vi "Begin.vi"(11 "Image Size":T1=enum."160x120") -> (0 "error out":errorcluster)   [LabVIEW 2012]
doc: "Called before other user functions, this VI is expected to open initial I/O refnums, load in file data, and do all program initialization. Notice that the <B>error out</B> terminal is simply used for data flow. Wiring it to other structures or subVIs ensures that this VI runs first."
uses:
  <vilib>/Rock Robotics/WPI/Camera/WPI_CameraImageSize.ctl
  <vilib>/Rock Robotics/SystemInterfaces/DIO/FPGA_DIOPWMChannel.ctl
  <vilib>/Rock Robotics/WPI/Camera/WPI_CameraWhite Balance Values.ctl
  <vilib>/Rock Robotics/WPI/Camera/WPI_CameraExposure Values.ctl
  <vilib>/Rock Robotics/WPI/Camera/WPI_CameraFrameRate.ctl
  <vilib>/Rock Robotics/WPI/SafetyOutput/WPI_SafetyOutputConfigMenu.ctl
  <vilib>/Rock Robotics/WPI/DriverStation/WPI_DriverStationRobotMode2.ctl
  <vilib>/Rock Robotics/WPI/Joystick/WPI_JoystickDeviceEnum.ctl
  <vilib>/Rock Robotics/SystemInterfaces/DIO/FPGA_DIORelayChannel.ctl
  <vilib>/Rock Robotics/SystemInterfaces/DIO/FPGA_DIOChannel.ctl
  <vilib>/Rock Robotics/WPI/Encoder/WPI_EncoderType.ctl
  <vilib>/Rock Robotics/SystemInterfaces/Typedef/FPGA_TypedefDigitalModule.ctl
  Program Files (x86)/National Instruments/LabVIEW 2012/examples/FRC/I2C/ADXL345 I2C/Driver/ADXL345 I2C Range.ctl
  <vilib>/Rock Robotics/WPI/RobotDrive/WPI_RobotDriveOpen2MotorWithJaguar.vi
  Robot Global Data.vi
  <vilib>/Rock Robotics/WPI/MotorControl/WPI_MotorControlOpen Jaguar.vi
  <vilib>/Rock Robotics/WPI/Counter/WPI_CounterDigitalInputToDigitalSource.vi
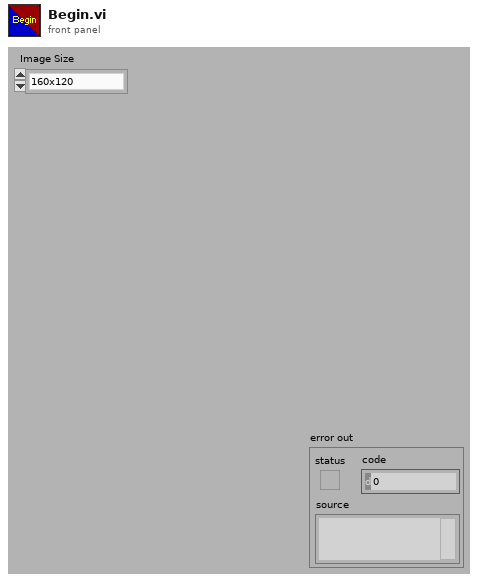
[diagram p1: front panel]
types:
  T1 = typedef "WPI_CameraImageSize.ctl" = enum16{"640x480", "320x240", "160x120"}
  T2 = typedef "FPGA_DIOPWMChannel.ctl" = enum8{"PWM 1", "PWM 2", "PWM 3", "PWM 4", "PWM 5", "PWM 6", "PWM 7", "PWM 8", "PWM 9", "PWM 10", "Invalid"}
  T3 = typedef "ADXL345 I2C Range.ctl" = u8
  T4 = typedef "FPGA_TypedefDigitalModule.ctl" = enum16{"Digital Module 1", "Digital Module 2"}
  T5 = typedef "WPI_EncoderType.ctl" = enum16{"1x", "2x", "4x"}
  T6 = typedef "FPGA_DIOChannel.ctl" = enum8{"DIO 1", "DIO 2", "DIO 3", "DIO 4", "DIO 5", "DIO 6", "DIO 7", "DIO 8", "DIO 9", "DIO 10", "DIO 11", "DIO 12", "DIO 13", "DIO 14", "Invalid"}
  T7 = typedef "FPGA_DIORelayChannel.ctl" = enum8{"Relay 1", "Relay 2", "Relay 3", "Relay 4", "Relay 5", "Relay 6", "Relay 7", "Relay 8", "Invalid"}
  T8 = typedef "WPI_JoystickDeviceEnum.ctl" = enum16{"USB 1", "USB 2", "USB 3", "USB 4", "Kinect 1", "Kinect 2"}
  T9 = typedef "WPI_DriverStationRobotMode2.ctl" = enum16{"Autonomous Disabled", "Autonomous Enabled", "Teleop Disabled", "Teleop Enabled", "Timeout", "Finish", "Test Disabled", "Test Enabled"}
  T10 = typedef "WPI_SafetyOutputConfigMenu.ctl" = enum16{"Enable", "Disable"}
  T11 = typedef "WPI_CameraFrameRate.ctl" = u32
  T12 = typedef "WPI_CameraExposure Values.ctl" = enum16{"Auto", "Flicker-free 50 Hz", "Flicker-free 60 Hz", "Hold current"}
  T13 = typedef "WPI_CameraWhite Balance Values.ctl" = enum16{"Auto", "Fixed indoor", "Fixed outdoor 1", "Fixed outdoor 2", "Fixed fluorescent 1", "Fixed fluorescent 2", "Hold current"}
  T14 = typedef "WPI_DigitalInputDevRef.ctl" = cluster{"DevStatus":errorcluster, "DIO Channel":T6, "Digital Module":T4}
  T15 = typedef "WPI_RelayDevRef.ctl" = cluster{"DevStatus":errorcluster, "Relay Channel":T7, "Digital Module":T4, "Relay Direction":T16}
  T16 = typedef "WPI_RelayDirection.ctl" = enum16{"Both directions", "Forward only", "Reverse only"}
  T17 = typedef "WPI_CameraDevRef.ctl" = cluster{"Camera Address":string, "CameraStatus":errorcluster, "Acquire Image Notifier":refnum<notifier>}
  T18 = typedef "WPI_JoystickDevRef.ctl" = cluster{"Device":T8}
  T19 = typedef "WPI_RobotDriveDevRef.ctl" = cluster{"DevStatus":errorcluster, "Motors[]":T20[], "Square Inputs":bool, "Max Output":dbl, "Isochronous":bool}
  T20 = typedef "WPI_MotorControlDeviceRef.ctl" = cluster{"DeviceStatus":errorcluster, "Type":enum16{"PWM", "CAN"}, "PWM":cluster{"Digital Module":T4, "PWM Channel":T2, "DeadBand":T21}, "CAN":cluster{"Device Number":u8, "Control Mode":T22, "Semaphore":T23, "Max Vout":dbl}, "Invert":bool, "TransformRef":T24, "InvTransformRef":T24}
  T21 = typedef "WPI_PWMDeadband.ctl" = cluster{"Name":string, "maxPositivePwm":i32, "minPositivePwm":i32, "centerPwm":i32, "maxNegativePwm":i32, "minNegativePwm":i32, "angularRange":u16}
  T22 = typedef "WPI_CANJaguar_ControlMode.ctl" = enum8{"Percent VBus", "Current", "Speed", "Position", "Voltage"}
  T23 = typedef "Semaphore RefNum" = refnum<k1>
  T24 = typedef "WPI_PWMTransform_ConPane.ctl" = refnum<vi>
  T25 = typedef "FPGA_CounterEncoderSourceConvertionLVSourceType.ctl" = cluster{"DevStatus":errorcluster, "AnalogTriggerMode?":bool, "DigitalMode":cluster{"Digital Module":T4, "DIO Channel":T26}, "AnalogTriggerMode":cluster{"AnalogTriggerIndex":T27, "OutputType":T28}}
  T26 = typedef "FPGA_DIODigitalSourceChannel.ctl" = enum8{"DIO 1", "DIO 2", "DIO 3", "DIO 4", "DIO 5", "DIO 6", "DIO 7", "DIO 8", "DIO 9", "DIO 10", "DIO 11", "DIO 12", "DIO 13", "DIO 14", "Disabled"}
  T27 = typedef "FPGA_AnalogTriggerIndex.ctl" = enum8{"Trig 0", "Trig 1", "Trig 2", "Trig 3", "Trig 4", "Trig 5", "Trig 6", "Trig 7", "Invalid"}
  T28 = typedef "FPGA_AnalogTriggerOutType.ctl" = enum16{"InWindow", "TriggerState", "Rising", "Falling"}
  T29 = typedef "WPI_I2CDevRef.ctl" = cluster{"DevStatus":errorcluster, "Digital Module":T4, "Device Address":u8}
  T30 = typedef "WPI_EncoderDevRef.ctl" = cluster{"DevStatus":errorcluster, "EncoderIndex":T31, "CounterIndex":T32, "DistancePerCount":dbl, "Decoding Type":T5}
  T31 = typedef "FPGA_EncoderIdx.ctl" = enum8{"Enc 0", "Enc 1", "Enc 2", "Enc 3", "Invalid"}
  T32 = typedef "FPGA_CounterCtrSystemIndex.ctl" = enum8{"Ctr 0", "Ctr 1", "Ctr 2", "Ctr 3", "Ctr 4", "Ctr 5", "Ctr 6", "Ctr 7", "Invalid"}
  T33 = typedef "WPI_ServoDeviceRef.ctl" = cluster{"DeviceStatus":errorcluster, "Digital Module":T4, "PWM Channel":T2, "DeadBand":T21}
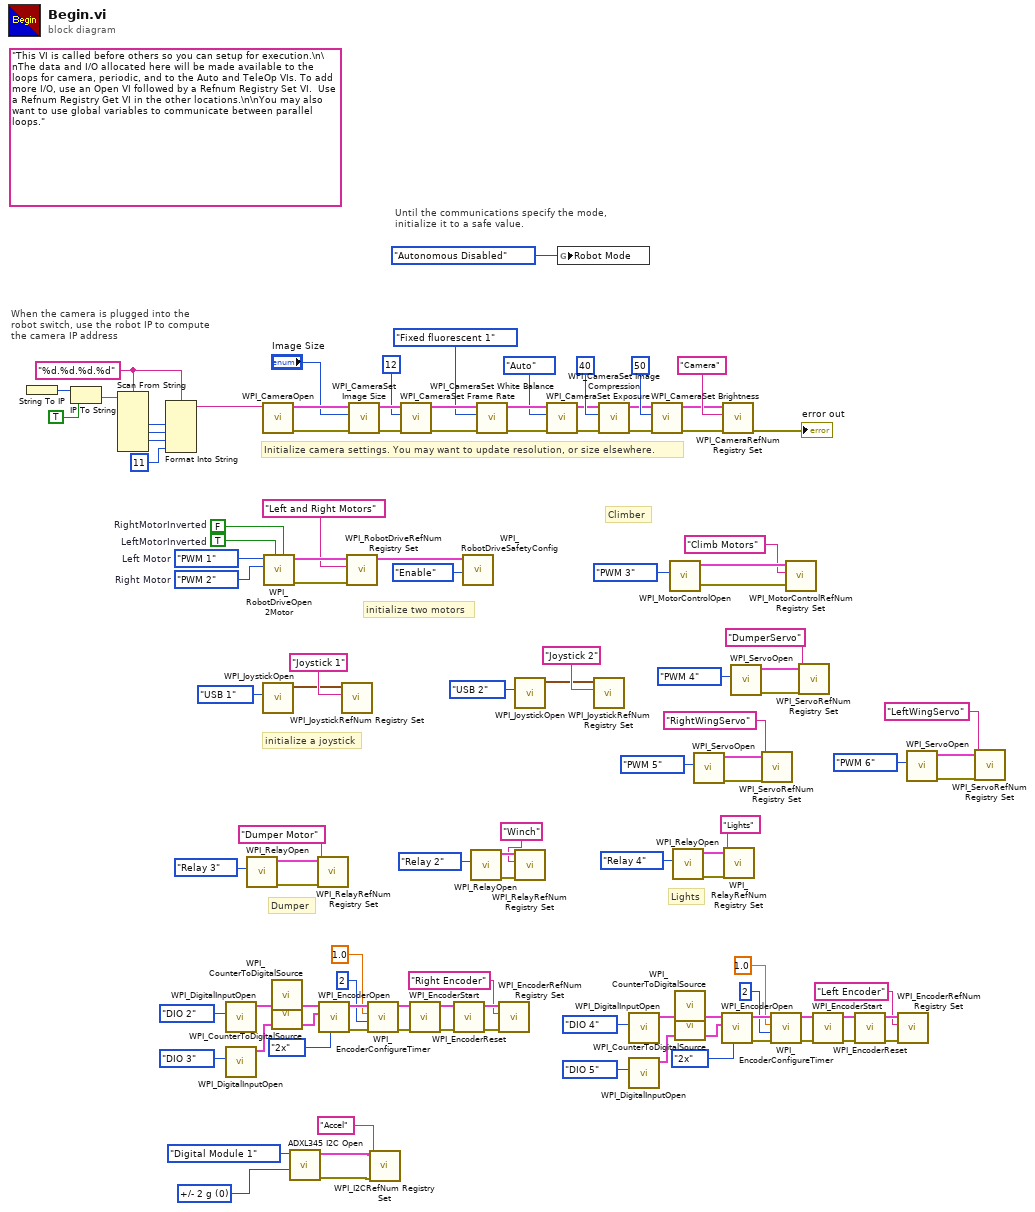
[diagram p0: block diagram]
diagram:
  w16 = T3 0 items=["+/- 2 g", "+/- 4 g", "+/- 8 g", "+/- 16 g"] ("Range")
  w81 = "%d.%d.%d.%d" ("format string")
  (unwired) "This VI is called before others so you can setup for execution.\n\nThe data and I/O allocated here will be made available to the loops for camera, periodic, and to the Auto and TeleOp VIs. To add more I/O, use an Open VI followed by a Refnum Registry Set VI.  Use a Refnum Registry Get VI in the other locations.\n\nYou may also want to use global variables to communicate between parallel loops."
  w92 = FPGA_DIOPWMChannel."PWM 2"  # Right Motor
  w93 = FPGA_DIOPWMChannel."PWM 1"  # Left Motor
  w115 = TRUE  # LeftMotorInverted
  w116 = FALSE  # RightMotorInverted
  # "Lights"
  # "Dumper"
  # "Climber"
  # "initialize a joystick"
  # "Until the communications specify the mode,\ninitialize it to a safe value."
  # "When the camera is plugged into the\nrobot switch, use the robot IP to compute\nthe camera IP address"
  # "initialize two motors"
  # "Initialize camera settings. You may want to update resolution, or size elsewhere."
  n1 = String To IP() -> (0:w88:u32)  [unwired: 1 in]
  n2 = IP To String(1:TRUE ("dot notation? (F)"), 2:w88) -> (0:w86:string)
  n3 = Scan From String(format string=w81, input string=w86) -> (output 1=w85:i32, output 2=w84:i32, output 3=w83:i32)  [unwired: 7 in, 3 out]
  n4 = Format Into String(format string=w81, w85, w84, w83, 11 ("Compression")) -> (resulting string=w77:string)  [unwired: 2 in, 1 out]
  n5 = call <vilib>:"WPI_DigitalInputOpen.vi"("DIO Channel"=FPGA_DIOChannel."DIO 2") -> ("DigitalInputDevRef"=w51:T14)  [unwired: 9 in, 1 out]
  n6 = call <vilib>:"WPI_DigitalInputOpen.vi"("DIO Channel"=FPGA_DIOChannel."DIO 3") -> ("DigitalInputDevRef"=w50:T14)  [unwired: 9 in, 1 out]
  n7 = call <vilib>:"WPI_RelayOpen.vi"("Relay Channel"=FPGA_DIORelayChannel."Relay 3") -> ("error out"=w62:errorcluster, "RelayDevRef"=w65:T15)  [unwired: 9 in]
  n8 = call <vilib>:"WPI_CameraOpen.vi"("Camera Address"=w77) -> ("error out"=w102:errorcluster, "CameraDevRef"=w103:T17)  [unwired: 1 in, 8 out]
  n9 = call <vilib>:"WPI_JoystickOpen.vi"("JoystickDevice"=WPI_JoystickDeviceEnum."USB 1") -> ("JoystickDevRef"=w75:T18)  [unwired: 10 in]
  n10 = call-poly <vilib>:"WPI_RobotDriveOpen2Motor.vi"("Right Motor Inverted"=w116, "Left Motor Inverted"=w115, "Right Motor"=w92, "Left Motor"=w93) -> ("error out"=w111:errorcluster, "RobotDriveDevRef"=w113:T19)  [unwired: 1 in, 5 out]
  n11 = call-poly <vilib>:"WPI_CounterToDigitalSource.vi"("DigitalInputDevRef"=w51) -> ("Digital Source"=w41:T25)  [unwired: 6 in]
  n12 = call-poly <vilib>:"WPI_CounterToDigitalSource.vi"("DigitalInputDevRef"=w50) -> ("Digital Source"=w40:T25)  [unwired: 6 in]
  n13 = call "ADXL345 I2C Open.vi"("Range"=w16, "DIO Module (Module 1)"=FPGA_TypedefDigitalModule."Digital Module 1") -> ("error out"=w14:errorcluster, "I2CDevRef"=w15:T29)  [unwired: 2 in, 6 out]
  n14 = call <vilib>:"WPI_RelayRefNum Registry Set.vi"("error in (no error)"=w62, "refnum name"="Dumper Motor", "RelayDevRef"=w65) -> ()  [unwired: 7 in, 2 out]
  n15 = call <vilib>:"WPI_EncoderOpen.vi"("Decoding Type"=WPI_EncoderType."2x", "BSource"=w40, "ASource"=w41) -> ("error out"=w49:errorcluster, "EncoderDevRef"=w45:T30)  [unwired: 7 in]
  n16 = call <vilib>:"WPI_JoystickRefNum Registry Set.vi"("refnum name"="Joystick 1", "JoystickDevRef"=w75) -> ()  [unwired: 8 in, 2 out]
  n17 = call <vilib>:"WPI_RobotDriveRefNum Registry Set.vi"("error in (no error)"=w111, "refnum name"="Left and Right Motors", "RobotDriveDevRef"=w113) -> ("RobotDriveDevRef"=w80:T19)  [unwired: 8 out]
  n18 = call <vilib>:"WPI_CameraSet Image Size.vi"("error in (no error)"=w102, "Image Size"="Image Size", "CameraDevRef"=w103) -> ("error out"=w101:errorcluster, "CameraDevRef Out"=w104:T17)  [unwired: 7 out]
  n19 = call <vilib>:"WPI_EncoderConfigureTimer.vi"("error in (no error)"=w49, "Number Samples to Average"=u8 2, "Minimum Rate"=1.0, "EncoderDevRef"=w45) -> ("error out"=w48:errorcluster, "EncoderDevRef"=w44:T30)  [unwired: 6 in]
  n20 = call <vilib>:"WPI_I2CRefNum Registry Set.vi"("error in (no error)"=w14, "refnum name"="Accel", "I2CDevRef"=w15) -> ()  [unwired: 7 in, 2 out]
  n21 = call <vilib>:"WPI_CameraSet Frame Rate.vi"("error in (no error)"=w101, "Frame Rate (fps)"=T11 12, "CameraDevRef"=w104) -> ("error out"=w100:errorcluster, "CameraDevRef Out"=w106:T17)  [unwired: 7 out]
  n22 = call <vilib>:"WPI_EncoderStart.vi"("error in (no error)"=w48, "EncoderDevRef"=w44) -> ("error out"=w47:errorcluster, "EncoderDevRef"=w43:T30)  [unwired: 8 in]
  n23 = call <vilib>:"WPI_EncoderReset.vi"("error in (no error)"=w47, "EncoderDevRef"=w43) -> ("error out"=w46:errorcluster, "EncoderDevRef"=w42:T30)  [unwired: 8 in]
  n24 = call <vilib>:"WPI_RobotDriveSafetyConfig.vi"("mode"=WPI_SafetyOutputConfigMenu."Enable", "RobotDriveDevRef"=w80) -> ()  [unwired: 8 in, 2 out]
  n25 = call <vilib>:"WPI_RelayOpen.vi"("Relay Channel"=FPGA_DIORelayChannel."Relay 2") -> ("error out"=w61:errorcluster, "RelayDevRef"=w60:T15)  [unwired: 9 in]
  n26 = call <vilib>:"WPI_CameraSet White Balance.vi"("error in (no error)"=w100, "White Balance"=WPI_CameraWhite_Balance_Values."Fixed fluorescent 1", "CameraDevRef"=w106) -> ("error out"=w99:errorcluster, "CameraDevRef Out"=w105:T17)  [unwired: 7 out]
  n27 = call <vilib>:"WPI_EncoderRefNum Registry Set.vi"("error in (no error)"=w46, "refnum name"="Right Encoder", "EncoderDevRef"=w42) -> ()  [unwired: 7 in, 2 out]
  n28 = call <vilib>:"WPI_JoystickOpen.vi"("JoystickDevice"=WPI_JoystickDeviceEnum."USB 2") -> ("JoystickDevRef"=w71:T18)  [unwired: 10 in]
  n29 = call <vilib>:"WPI_RelayRefNum Registry Set.vi"("error in (no error)"=w61, "refnum name"="Winch", "RelayDevRef"=w60) -> ()  [unwired: 7 in, 2 out]
  n30 = call <vilib>:"WPI_CameraSet Exposure.vi"("error in (no error)"=w99, "Exposure"=WPI_CameraExposure_Values."Auto", "CameraDevRef"=w105) -> ("error out"=w98:errorcluster, "CameraDevRef Out"=w108:T17)  [unwired: 7 out]
  n31 = global write "Robot Global Data.vi" "Robot Mode"(WPI_DriverStationRobotMode2."Autonomous Disabled" ("Robot Mode")) -> ()
  n32 = call <vilib>:"WPI_JoystickRefNum Registry Set.vi"("refnum name"="Joystick 2", "JoystickDevRef"=w71) -> ()  [unwired: 8 in, 2 out]
  n33 = call <vilib>:"WPI_CameraSet Image Compression.vi"("error in (no error)"=w98, "Compression"=40, "CameraDevRef"=w108) -> ("error out"=w97:errorcluster, "CameraDevRef Out"=w107:T17)  [unwired: 7 out]
  n34 = call <vilib>:"WPI_DigitalInputOpen.vi"("DIO Channel"=FPGA_DIOChannel."DIO 4") -> ("DigitalInputDevRef"=w34:T14)  [unwired: 9 in, 1 out]
  n35 = call <vilib>:"WPI_DigitalInputOpen.vi"("DIO Channel"=FPGA_DIOChannel."DIO 5") -> ("DigitalInputDevRef"=w18:T14)  [unwired: 9 in, 1 out]
  n36 = call <vilib>:"WPI_CameraSet Brightness.vi"("error in (no error)"=w97, "Brightness"=50, "CameraDevRef"=w107) -> ("error out"=w95:errorcluster, "CameraDevRef Out"=w96:T17)  [unwired: 7 out]
  n37 = call-poly <vilib>:"WPI_MotorControlOpen.vi"("PWM Channel"=FPGA_DIOPWMChannel."PWM 3") -> ("error out"=w67:errorcluster, "MotorControlDeviceRef"=w69:T20)  [unwired: 9 in]
  n38 = call <vilib>:"WPI_RelayOpen.vi"("Relay Channel"=FPGA_DIORelayChannel."Relay 4") -> ("error out"=w56:errorcluster, "RelayDevRef"=w57:T15)  [unwired: 9 in]
  n39 = call-poly <vilib>:"WPI_CounterToDigitalSource.vi"("DigitalInputDevRef"=w34) -> ("Digital Source"=w25:T25)  [unwired: 6 in]
  n40 = call-poly <vilib>:"WPI_CounterToDigitalSource.vi"("DigitalInputDevRef"=w18) -> ("Digital Source"=w24:T25)  [unwired: 6 in]
  n41 = call <vilib>:"WPI_ServoOpen.vi"("PWM Channel"=FPGA_DIOPWMChannel."PWM 5") -> ("error out"=w6:errorcluster, "ServoDeviceRef"=w8:T33)  [unwired: 9 in]
  n42 = call <vilib>:"WPI_EncoderOpen.vi"("Decoding Type"=WPI_EncoderType."2x", "BSource"=w24, "ASource"=w25) -> ("error out"=w33:errorcluster, "EncoderDevRef"=w29:T30)  [unwired: 7 in]
  n43 = call <vilib>:"WPI_CameraRefNum Registry Set.vi"("error in (no error)"=w95, "refnum name"="Camera", "CameraDevRef"=w96) -> ("error out"=→"error out":errorcluster)  [unwired: 8 out]
  n44 = call <vilib>:"WPI_RelayRefNum Registry Set.vi"("error in (no error)"=w56, "refnum name"="Lights", "RelayDevRef"=w57) -> ()  [unwired: 7 in, 2 out]
  n45 = call <vilib>:"WPI_ServoOpen.vi"("PWM Channel"=FPGA_DIOPWMChannel."PWM 4") -> ("error out"=w10:errorcluster, "ServoDeviceRef"=w12:T33)  [unwired: 9 in]
  n46 = call <vilib>:"WPI_ServoRefNum Registry Set.vi"("error in (no error)"=w6, "refnum name"="RightWingServo", "ServoDeviceRef"=w8) -> ()  [unwired: 7 in, 2 out]
  n47 = call <vilib>:"WPI_EncoderConfigureTimer.vi"("error in (no error)"=w33, "Number Samples to Average"=u8 2, "Minimum Rate"=1.0, "EncoderDevRef"=w29) -> ("error out"=w32:errorcluster, "EncoderDevRef"=w28:T30)  [unwired: 6 in]
  n48 = call <vilib>:"WPI_MotorControlRefNum Registry Set.vi"("error in (no error)"=w67, "refnum name"="Climb Motors", "MotorControlDevRef"=w69) -> ()  [unwired: 7 in, 2 out]
  n49 = call <vilib>:"WPI_ServoRefNum Registry Set.vi"("error in (no error)"=w10, "refnum name"="DumperServo", "ServoDeviceRef"=w12) -> ()  [unwired: 7 in, 2 out]
  n50 = call <vilib>:"WPI_EncoderStart.vi"("error in (no error)"=w32, "EncoderDevRef"=w28) -> ("error out"=w31:errorcluster, "EncoderDevRef"=w27:T30)  [unwired: 8 in]
  n51 = call <vilib>:"WPI_EncoderReset.vi"("error in (no error)"=w31, "EncoderDevRef"=w27) -> ("error out"=w30:errorcluster, "EncoderDevRef"=w26:T30)  [unwired: 8 in]
  n52 = call <vilib>:"WPI_EncoderRefNum Registry Set.vi"("error in (no error)"=w30, "refnum name"="Left Encoder", "EncoderDevRef"=w26) -> ()  [unwired: 7 in, 2 out]
  n53 = call <vilib>:"WPI_ServoOpen.vi"("PWM Channel"=FPGA_DIOPWMChannel."PWM 6") -> ("error out"=w2:errorcluster, "ServoDeviceRef"=w4:T33)  [unwired: 9 in]
  n54 = call <vilib>:"WPI_ServoRefNum Registry Set.vi"("error in (no error)"=w2, "refnum name"="LeftWingServo", "ServoDeviceRef"=w4) -> ()  [unwired: 7 in, 2 out]
